vi "Get Tx Generic Command Section and Channels.vi"(8 "error in":errorcluster, 11 "Tx generic ref":T1 format="%.0x") -> (0 "error out":errorcluster, 1 "Tx generic command channel refs":T1[](array[typedef]) format="%.0x", 2 "Tx generic command section ref out":T1 format="%.0x", 3 "Tx generic ref out":T1 format="%.0x", 4 "found?":bool)   [LabVIEW 2020, in "AIM ARINC 664 Scripting.lvlib"]
uses:
  AIM ARINC 664 Scripting.lvlib
  <vilib>/NI VeriStand/Custom Device API/Custom Device Item Ref.ctl
  Constants.vi
  <vilib>/NI VeriStand/Custom Device API/Custom Device API.lvlib
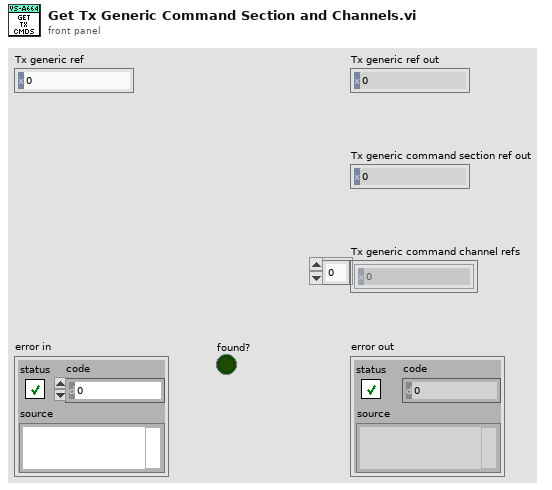
[diagram p1: front panel]
types:
  T1 = typedef "Custom Device API.lvlib/Custom Device Item Ref.ctl" = u64
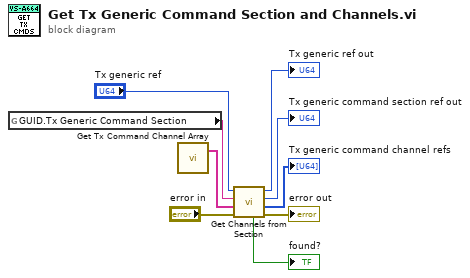
[diagram p0: block diagram]
diagram:
  n1 = global read "Constants.vi" "GUID.Tx Generic Command Section"() -> (w9:string)
  n2 = call "Get Tx Command Channel Array.vi"() -> ("Channel Array"=w8:string[])  [unwired: 3 in]
  n3 = call "Get Channels from Section.vi"("error in"="error in", "channel array names"=w8, "GUID section"=w9, "custom device ref in"="Tx generic ref") -> ("error out"=→"error out":errorcluster, "channel array refs out"=→"Tx generic command channel refs":T1[], "section ref out"=→"Tx generic command section ref out":T1, "custom device ref out"=→"Tx generic ref out":T1, "all channels found?"=→"found?":bool)  [unwired: 2 in, 1 out]
